vi "FMDLClusterToHeaderBlock.vi"() -> ()   [LabVIEW 2018]
panel:
  out "error out":errorcluster
  in  "error in (no error)":errorcluster
  in  "Voltage bias settings":T1={"Steps (number)"=101, "Vdevice (starting, V)"=0.0, "Vdevice (ending, V)"=10.0, "Measurement speed (PLC)"=1.0, "High capacitance?"=FALSE, "Accurate readback?"=TRUE, "Current compliance (A)"=1.0, "Number of readings to average/measurement"=1} {"Number of readings to average/measurement" items=["1"=1, "10"=10, "50"=50]; "Vdevice (ending, V)" min=0.1 max=12.0 step=0.05; "Vdevice (starting, V)" min=0.0 max=20.0 step=0.05; "Steps (number)" min=5 max=1001 step=1}
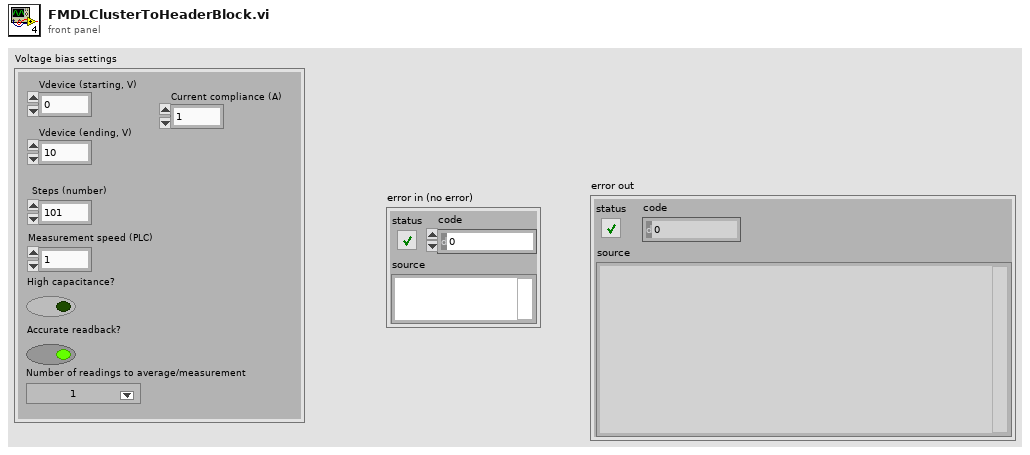
[diagram p1: front panel]
types:
  T1 = cluster{"Steps (number)":i32, "Vdevice (starting, V)":dbl, "Vdevice (ending, V)":dbl, "Measurement speed (PLC)":dbl, "High capacitance?":bool, "Accurate readback?":bool, "Current compliance (A)":dbl, "Number of readings to average/measurement":u16}
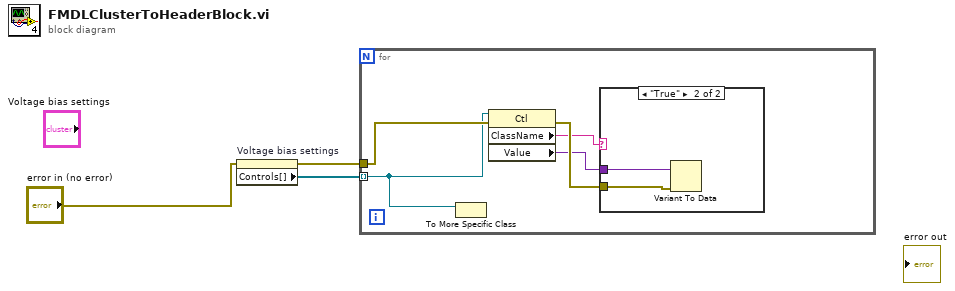
[diagram p0: block diagram]
diagram:
  n1 = property on="Voltage bias settings" class="Clust (strict)"(error in="error in (no error)") -> (error out=w1:errorcluster, "Controls[]"=w2:refnum<vi>[])  [unwired: 1 in, 1 out]
  n2 = for {
    tunnel: w2 -> [w4] mode=indexing
    tunnel: w1 -> [w8]
    n3 = To More Specific Class(reference=w4) -> ()  [unwired: 2 in, 2 out]
    n4 = property class="Ctl"(reference=w4, error in=w8) -> (error out=w7:errorcluster, "ClassName"=w6:string, "Value"=w5:variant)  [unwired: 1 out]
    n5 = case shown="\"True\"" w6 {
      tunnel: w5 -> [_ w10]
      tunnel: w7 -> [_ w9]
      frame "False", Default {
      }
      frame "True" {
        n6 = Variant To Data(error in=w9, Variant=w10) -> ()  [unwired: 1 in, 2 out]
      }
    }
  }
